vi "_TangoStateColor.vi"(1 "State":T1) -> (0 "State Color":u32(colorbox)=16448250)   [LabVIEW 2014, in "tango.lvlib"]
uses:
  tango.lvlib
  Typedefs/_TangoState_t.ctl
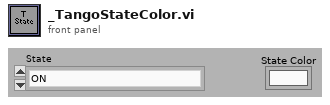
[diagram p1: front panel]
types:
  T1 = typedef "tango.lvlib/_TangoState_t.ctl" = enum32{"ON", "OFF", "CLOSE", "OPEN", "INSERT", "EXTRACT", "MOVING", "STANDBY", "FAULT", "INIT", "RUNNING", "ALARM", "DISABLE", "UNKNOWN"}
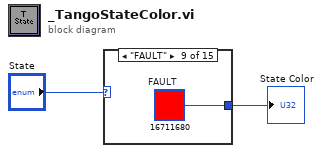
[diagram p0: block diagram]
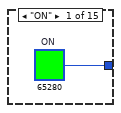
[diagram p2: hidden frame]
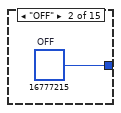
[diagram p3: hidden frame]
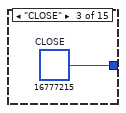
[diagram p4: hidden frame]
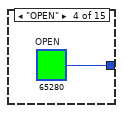
[diagram p5: hidden frame]
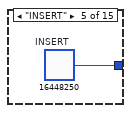
[diagram p6: hidden frame]
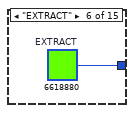
[diagram p7: hidden frame]
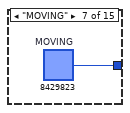
[diagram p8: hidden frame]
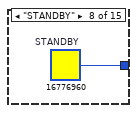
[diagram p9: hidden frame]
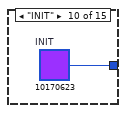
[diagram p10: hidden frame]
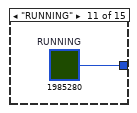
[diagram p11: hidden frame]
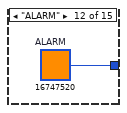
[diagram p12: hidden frame]
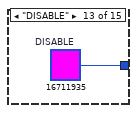
[diagram p13: hidden frame]
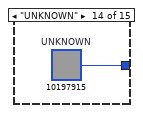
[diagram p14: hidden frame]
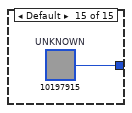
[diagram p15: hidden frame]
diagram:
  n1 = case shown="\"FAULT\"" "State" {
    tunnel: [w3 w4 w5 w6 w7 w8 w9 w10 w11 w12 w13 w14 w15 w16 w17] -> w2
    frame "ON" {
      w3 = u32 65280  # ON
    }
    frame "OFF" {
      w4 = u32 16777215  # OFF
    }
    frame "CLOSE" {
      w5 = u32 16777215  # CLOSE
    }
    frame "OPEN" {
      w6 = u32 65280  # OPEN
    }
    frame "INSERT" {
      w7 = u32 16448250  # INSERT
    }
    frame "EXTRACT" {
      w8 = u32 6618880  # EXTRACT
    }
    frame "MOVING" {
      w9 = u32 8429823  # MOVING
    }
    frame "STANDBY" {
      w10 = u32 16776960  # STANDBY
    }
    frame "FAULT" {
      w11 = u32 16711680  # FAULT
    }
    frame "INIT" {
      w12 = u32 10170623  # INIT
    }
    frame "RUNNING" {
      w13 = u32 1985280  # RUNNING
    }
    frame "ALARM" {
      w14 = u32 16747520  # ALARM
    }
    frame "DISABLE" {
      w15 = u32 16711935  # DISABLE
    }
    frame "UNKNOWN" {
      w16 = u32 10197915  # UNKNOWN
    }
    frame Default {
      w17 = u32 10197915  # UNKNOWN
    }
  }
  "State Color" <- w2
